vi "Get Cell Values.vi"(7 "Sheet Name":string, 8 "error in":errorcluster, 10 "Cell Addresses":string="A1:B1", 11 "SpreadsheetDoc in":refnum<k24>) -> (0 "error out":errorcluster, 1 "Types":T1[][](array[typedef]), 2 "Cell Values":T2(array[cluster]) {"Time Stamp" format="%<%x %.3X>T"}, 3 "SpreadsheetDoc out":refnum<k24>)   [LabVIEW 2019, in "Open Xml.lvlib"]
uses:
  Open Xml.lvlib
  D:/git/Open-Xml-LabVIEW/Source/DocumentFormat.OpenXml.dll
  DocumentFormat.OpenXml.dll
  Cell DataType.ctl
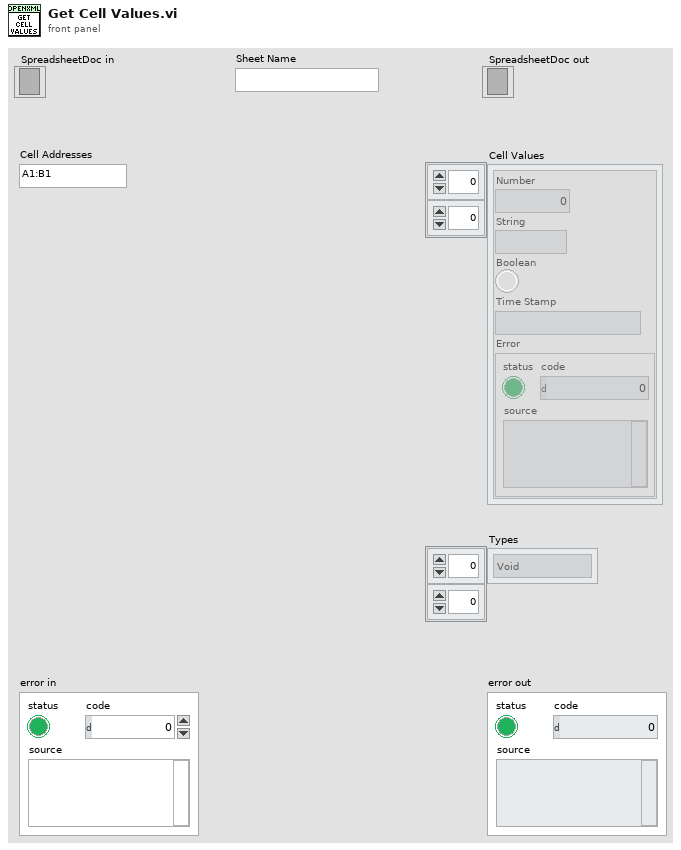
[diagram p1: front panel]
types:
  T1 = typedef "Open Xml.lvlib/Cell DataType.ctl" = enum16{"Void", "Boolean", "Number", "Error", "SharedString", "String", "InlineString", "Date"}
  T2 = cluster{"Number":dbl, "String":string, "Boolean":bool, "Time Stamp":timestamp, "Error":errorcluster}[][]
  T3 = cluster{"Number":dbl, "String":string, "Boolean":bool, "Time Stamp":timestamp, "Error":errorcluster}
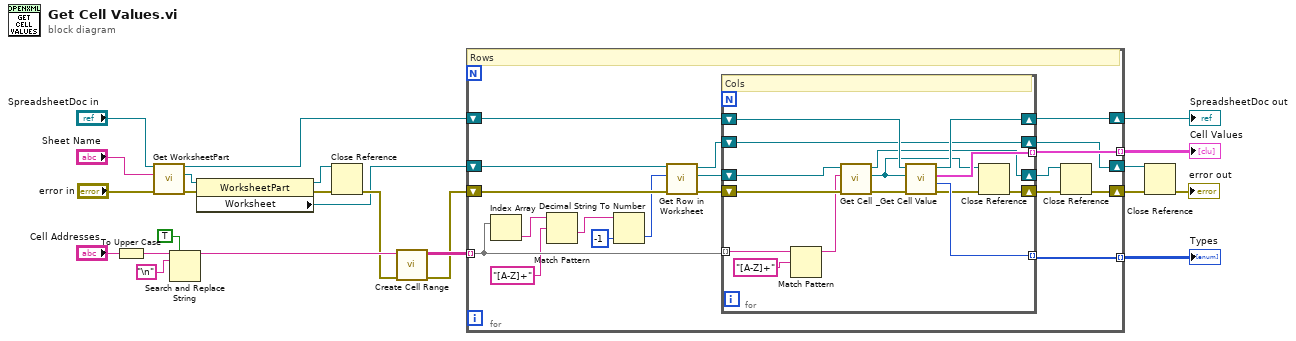
[diagram p0: block diagram]
diagram:
  n1 = To Upper Case(1:"Cell Addresses") -> (0:w11:string)
  n2 = call "Get WorksheetPart.vi"("error in"="error in", "Sheet Name"="Sheet Name", "SpreadsheetDocument in"="SpreadsheetDoc in") -> ("error out"=w6:errorcluster, "WorksheetPart"=w5:refnum<k24>, "SpreadsheetDocument out"=w17:refnum<k24>)  [unwired: 6 in]
  n3 = Search and Replace String(replace all?=TRUE ("replace all? (F)"), input string=w11, search string="\n") -> (result string=w10:string)  [unwired: 5 in, 3 out]
  n4 = property class="WorksheetPart"(reference=w5, error in=w6) -> (reference out=w2:refnum<k24>, error out=w4:errorcluster, "Worksheet"=w1:refnum<k24>)
  n5 = Close Reference(reference=w2, error in (no error)=w4) -> (error out=w3:errorcluster)
  n6 = call "Create Cell Range.vi"("error in"=w3, "Cell Range"=w10) -> ("error out"=w13:errorcluster, "Cell Range"=w20:string[][])  [unwired: 8 in]
  n7 = for {
    tunnel: w20 -> [w32] mode=indexing
    tunnel: [w39] -> w16 mode=indexing
    tunnel: [w38] -> w15 mode=indexing
    shift-right: [w41] -> w21
    shift-left: w17 -> [w40]
    shift-right: [w25] -> w22
    shift-left: w13 -> [w36]
    shift-right: [w37] -> w14
    shift-left: w1 -> [w34]
    # "Rows"
    n8 = Index Array(array=w32) -> (element=w31:string)  [unwired: 1 in]
    n9 = Match Pattern(string=w31, regular expression="[A-Z]+") -> (after substring=w28:string)  [unwired: 1 in, 3 out]
    n10 = Decimal String To Number(string=w28, default (0L)=-1 ("default (0 I32)")) -> (number=w27:i32)  [unwired: 1 in, 1 out]
    n11 = call "Get Row in Worksheet.vi"("error in"=w36, "RowIndex"=w27, "Worksheet in"=w34) -> ("error out"=w35:errorcluster, "Row out"=w26:refnum<k24>, "Worksheet out"=w33:refnum<k24>)  [unwired: 6 in]
    n12 = for {
      tunnel: [w52] -> w39 mode=indexing
      tunnel: [w51] -> w38 mode=indexing
      shift-right: [w55] -> w42
      shift-left: w35 -> [w56]
      shift-right: [w53] -> w41
      shift-left: w40 -> [w54]
      tunnel: w32 -> [w46] mode=indexing
      shift-right: [w43] -> w24
      shift-left: w26 -> [w44]
      shift-right: [w45] -> w37
      shift-left: w33 -> [w45]
      # "Cols"
      n13 = Match Pattern(string=w46, regular expression="[A-Z]+") -> ()  [unwired: 1 in, 4 out]
      n14 = call "Get Cell.vi"("error in"=w56, "Cell Address"=w46, "Row in"=w44) -> ("error out"=w50:errorcluster, "Cell"=w48:refnum<k24>, "Row out"=w43:refnum<k24>)  [unwired: 6 in]
      n15 = call "_Get Cell Value.vi"("error in"=w50, "Cell"=w48, "SpreadsheetDoc in"=w54) -> ("error out"=w49:errorcluster, "Type"=w51:T1, "Cell Value"=w52:T3, "SpreadsheetDocument out"=w53:refnum<k24>)  [unwired: 5 in]
      n16 = Close Reference(reference=w48, error in (no error)=w49) -> (error out=w55:errorcluster)
    }
    n17 = Close Reference(reference=w24, error in (no error)=w42) -> (error out=w25:errorcluster)
  }
  "SpreadsheetDoc out" <- w21
  "Cell Values" <- w16
  "Types" <- w15
  n18 = Close Reference(reference=w14, error in (no error)=w22) -> (error out=→"error out":errorcluster)
